vi "pp2_webcam_test_assistantB.vi"(0 "Focus::Mode":u32(ring)=1 items=["Auto"=1, "Manual"=2], 5 "Stop (F)":bool, 7 "error in":errorcluster) -> (20 "Image Out":T1(plugin-control), 22 "Image Number":u32, 24 "Stopped":bool, 25 "Frame Rate":dbl, 26 "Image Logging Path Out":path, 27 "error out":errorcluster)   [LabVIEW 2013]
doc: "Creates, and edits acquisitions using the NI Vision Acquisition Express VI.\n\nThe NI Vision Acquisition Wizard is launched by placing the Express VI on the block diagram. Select an acquisition source and configure an acquisition using NI-IMAQ, NI-IMAQdx, or simulate an acquisition by reading an AVI or image files from a folder. After an acquisition is configured, select controls and indicators to be able to programmatically set in LabVIEW. Double-click the Vision Acquisition Express VI to edit the acquisition.\n\nNote: Any images created by the Express VI need to be disposed after use. Use the IMAQ Dispose.vi to cleanup the images output by the Express VI when they are no longer needed."
uses:
  <vilib>/vision/driver/Vision Acquisition Express Utility VIs.llb/Vision Acquisition Path Convert (String).vi
  <vilib>/vision/driver/NI_Vision_Acquisition_Software.lvlib
  <resource>/objmgr/imaqdx.rc
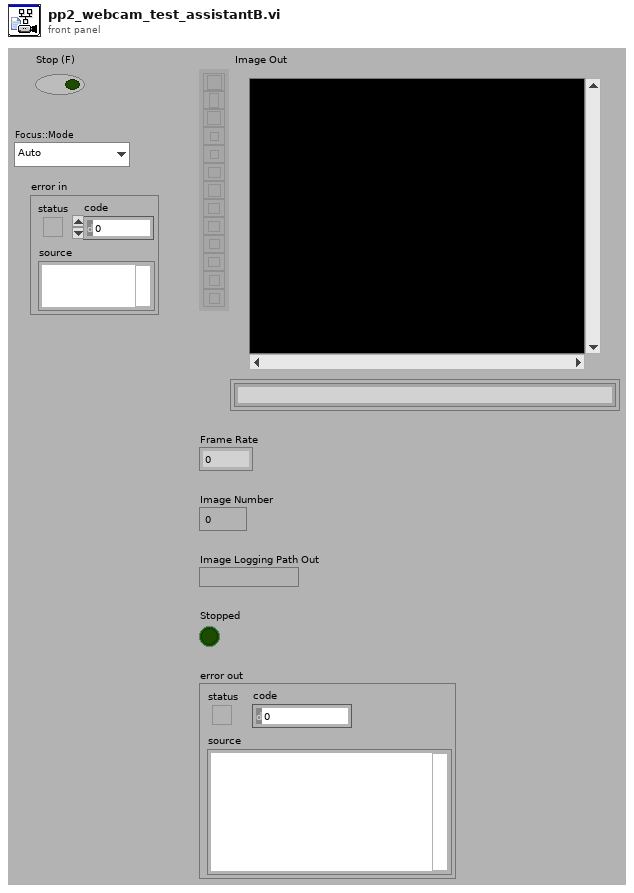
[diagram p1: front panel]
types:
  T1 = typedef "IMAQ Image.ctl" = refnum<image>
  T2 = typedef "IMAQdx.ctl" = refnum<k21>
  T3 = cluster{"File Type":string, "Quality":u32, "Compress":bool, "Lossless":bool, "Ratio":sgl, "Codec":string, "Frame Rate":u32, "Limit Frames":bool, "Max Frames":u32}
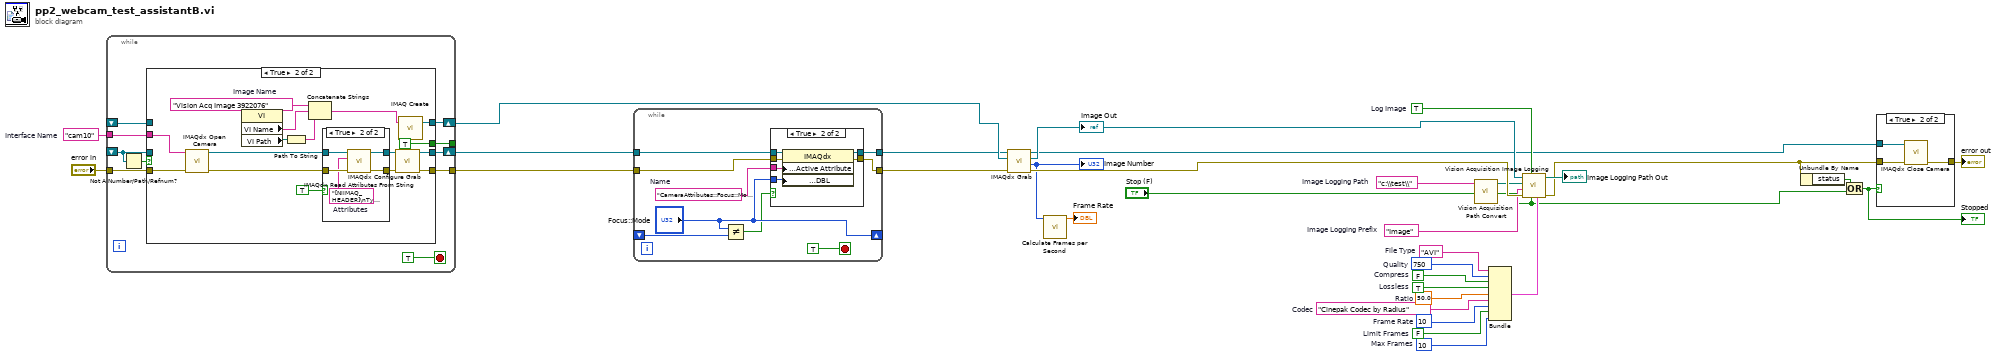
[diagram p0: block diagram]
diagram:
  w6 = "c:\\test\\"  # Image Logging Path
  w9 = TRUE  # Log Image
  w20 = "Image"  # Image Logging Prefix
  w15 = sgl 50.0  # Ratio
  w16 = TRUE  # Lossless
  w17 = FALSE  # Compress
  w18 = u32 750  # Quality
  w14 = "Cinepak Codec by Radius"  # Codec
  w13 = u32 10  # Frame Rate
  w11 = u32 10  # Max Frames
  w12 = FALSE  # Limit Frames
  w19 = "AVI"  # File Type
  w30 = "cam10"  # Interface Name
  n1 = while "While Loop_template0" {
    shift-right: [w42] -> w29
    shift-left: _ -> [w35]
    tunnel: [w41] -> w31
    tunnel: "error in" -> [w40]
    shift-right: [w38] -> w27
    shift-left: _ -> [w37]
    tunnel: w30 -> [w36]
    tunnel: [w33] -> _
    stop <- TRUE ("_template0") stop-if-true
    n2 = Not A Number/Path/Refnum?(number/path/refnum=w35) -> (NaN/Path/Refnum?=w34:bool)
    n3 = case "Case Structure_template0" shown="True" w34 {
      tunnel: [w45 w60] -> w42
      tunnel: w35 -> [w45 _]
      tunnel: [w44 w59] -> w41
      tunnel: w40 -> [w44 w61]
      tunnel: [w43 w58] -> w38
      tunnel: w37 -> [w43 _]
      tunnel: w36 -> [_ w48]
      tunnel: [_ TRUE] -> w33
      frame False {
      }
      frame True {
        w53 = "Vision Acq Image 3922076"  # Image Name
        n4 = call <vilib>:"IMAQdx Open Camera.vi"("error in"=w61, "Session In"=w48) -> ("error out"=w51:errorcluster, "Session Out"=w52:T2)  [unwired: 1 in, 7 out]
        n5 = property class="VI"() -> ("VI Name"=w56:string, "VI Path"=w57:path)  [unwired: 2 in, 2 out]
        n6 = Path To String(path=w57) -> (string=w55:string)
        n7 = Concatenate Strings(w53, w56, w55) -> (w54:string)
        n8 = case shown="True" TRUE ("Init Attributes") {
          tunnel: w52 -> [w63 w68]
          tunnel: w51 -> [w62 w67]
          tunnel: [w63 w65] -> w50
          tunnel: [w62 w64] -> w49
          frame False {
          }
          frame True {
            w66 = "[NIIMAQ_HEADER]\nType = 2\nVersion = 8\n\n[CAMERA_DATA]\nAcquisitionAttributes::Bayer::Algorithm = \"Bilinear\"\nAcquisitionAttributes::Bayer::GainB = \"1\"\nAcquisitionAttributes::Bayer::GainG = \"1\"\nAcquisitionAttributes::Bayer::GainR = \"1\"\nAcquisitionAttributes::Bayer::Pattern = \"Use hardware value\"\nAcquisitionAttributes::BitsPerPixel = \"Use hardware value\"\nAcquisitionAttributes::IgnoreFirstFrame = \"false\"\nAcquisitionAttributes::ImageDecoderCopyMode = \"Auto\"\nAcquisitionAttributes::OutputImageType = \"Auto\"\nAcquisitionAttributes::OverwriteMode = \"Get Newest\"\nAcquisitionAttributes::PixelSignedness = \"Use hardware value\"\nAcquisitionAttributes::ReceiveTimestampMode = \"None\"\nAcquisitionAttributes::ShiftPixelBits = \"false\"\nAcquisitionAttributes::SwapPixelBytes = \"false\"\nAcquisitionAttributes::Timeout = \"5000\"\nAcquisitionAttributes::VerticalMirror = \"false\"\nAcquisitionAttributes::VideoMode = \"800x448 RGB24 30.00fps\"\nCameraAttributes::BacklightCompensation::Mode = \"Manual\"\nCameraAttributes::BacklightCompensation::Value = \"false\"\nCameraAttributes::Brightness::Mode = \"Manual\"\nCameraAttributes::Brightness::Value = \"133\"\nCameraAttributes::Contrast::Mode = \"Manual\"\nCameraAttributes::Contrast::Value = \"0.050000000000000003\"\nCameraAttributes::Exposure::Mode = \"Auto\"\nCameraAttributes::Focus::Mode = \"Auto\"\nCameraAttributes::Pan::Mode = \"Manual\"\nCameraAttributes::Pan::Value = \"0\"\nCameraAttributes::Saturation::Mode = \"Manual\"\nCameraAttributes::Saturation::Value = \"83\"\nCameraAttributes::Sharpness::Mode = \"Manual\"\nCameraAttributes::Sharpness::Value = \"20\"\nCameraAttributes::Tilt::Mode = \"Manual\"\nCameraAttributes::Tilt::Value = \"0\"\nCameraAttributes::WhiteBalance::Mode = \"Auto\"\nCameraAttributes::Zoom::Mode = \"Manual\"\nCameraAttributes::Zoom::Value = \"0\"\n"  # Attributes
            n9 = call <vilib>:"IMAQdx Read Attributes From String.vi"("error in"=w67, "Attributes String In"=w66, "Session In"=w68) -> ("error out"=w64:errorcluster, "Session Out"=w65:T2)  [unwired: 7 out]
          }
        }
        n10 = call <vilib>:"IMAQdx Configure Grab.vi"("error in"=w49, "Session In"=w50) -> ("error out"=w59:errorcluster, "Session Out"=w60:T2)  [unwired: 8 out]
        n11 = call "IMAQ Create"("Image Name"=w54) -> ("New Image"=w58:T1)  [unwired: 3 in, 2 out]
      }
    }
  }
  n12 = while {
    tunnel: w31 -> [w77]
    tunnel: [w76] -> w26
    tunnel: w29 -> [w75]
    tunnel: [w74] -> w28
    shift-right: ["Focus::Mode"] -> _
    shift-left: _ -> [w70]
    stop <- TRUE stop-if-true
    w73 = "CameraAttributes::Focus::Mode"  # Name
    n13 = Not Equal?(x="Focus::Mode", y=w70) -> (x != y?=w69:bool)
    n14 = case shown="True" w69 {
      tunnel: w77 -> [w78 w85]
      tunnel: [w79 w84] -> w76
      tunnel: w75 -> [w79 w83]
      tunnel: [w78 w82] -> w74
      tunnel: w73 -> [_ w81]
      tunnel: "Focus::Mode" -> [_ w80]
      frame False {
      }
      frame True {
        n15 = property class="IMAQdx"(reference=w83, error in=w85, "Camera Attributes:Active Attribute"=w81, "Camera Attributes:Value:DBL"=w80) -> (reference out=w84:T2, error out=w82:errorcluster)
      }
    }
  }
  n16 = call <vilib>:"IMAQdx Grab.vi"("error in"=w28, "Image In"=w27, "Session In"=w26) -> ("error out"=w25:errorcluster, "Buffer Number Out"=w24:u32, "Image Out"=w21:T1, "Session Out"=w5:T2)  [unwired: 1 in, 4 out]
  "Image Out" <- w21
  "Image Number" <- w24
  n17 = call <vilib>:"Calculate Frames per Second.vi"("Buffer Number"=w24) -> ("Acquired Frames/s"=→"Frame Rate":dbl)  [unwired: 2 in, 8 out]
  n18 = call-poly <vilib>:"Vision Acquisition Path Convert.vi"("Path In"=w6) -> ("Path Out"=w7:path)  [unwired: 10 in]
  n19 = Bundle("File Type"=w19, "Quality"=w18, "Compress"=w17, "Lossless"=w16, "Ratio"=w15, "Codec"=w14, "Frame Rate"=w13, "Limit Frames"=w12, "Max Frames"=w11) -> (w8:T3)  [unwired: 1 out]
  n20 = call <vilib>:"Vision Acquisition Image Logging.vi"("File Settings"=w8, "Close"="Stop (F)", "Log Image"=w9, "error in (no error)"=w25, "Image Logging Prefix"=w20, "Image Logging Path"=w7, "Image In"=w21) -> ("error out"=w10:errorcluster, "Image Logging Path Out"=→"Image Logging Path Out":path)  [unwired: 3 out]
  n21 = Unbundle By Name(w10) -> ("status"=w1:bool)
  n22 = Or(x=w1, y="Stop (F)") -> (x .or. y?=w2:bool)
  "Stopped" <- w2
  n23 = case "Case Structure_template1" shown="True" w2 {
    tunnel: [w86 w88] -> w4
    tunnel: w10 -> [w86 w89]
    tunnel: w5 -> [_ w87]
    frame False {
    }
    frame True {
      n24 = call <vilib>:"IMAQdx Close Camera.vi"("error in"=w89, "Session In"=w87) -> ("error out"=w88:errorcluster)  [unwired: 9 out]
    }
  }
  "error out" <- w4
